vi "Destroy UI Events.vi"(11 "Process in":refnum<class "ABD.lvclass">) -> ()   [LabVIEW 2021, in "ABD.lvlib" / "ABD.lvclass"]
uses:
  ABD.lvclass
  ABD.lvclass/ABD.ctl
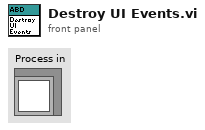
[diagram p1: front panel]
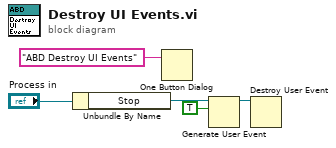
[diagram p0: block diagram]
diagram:
  n1 = Unbundle By Name("Process in") -> ("Stop"=w4:refnum<user-event>)
  n2 = One Button Dialog(message="ABD Destroy UI Events") -> ()  [unwired: 1 in, 1 out]
  n3 = Generate User Event(user event=w4, event data cluster=TRUE ("event data")) -> (user event out=w3:refnum<user-event>)  [unwired: 2 in, 1 out]
  n4 = Destroy User Event(user event=w3) -> ()  [unwired: 1 in, 1 out]
